vi "test_Outgoing2 Waveforms.vi"(8 "error in (no error)":errorcluster, 11 "DMA Channels Basic Testing in":refnum<class "FPGA Addon DMA Channels Interleaved System Tests.lvclass">) -> (0 "error out":errorcluster, 3 "DMA Channels Basic Testing out":refnum<class "FPGA Addon DMA Channels Interleaved System Tests.lvclass">)   [LabVIEW 2020, in "FPGA Addon DMA Channels Interleaved System Tests.lvclass"]
uses:
  FPGA Addon DMA Channels Interleaved System Tests.lvclass
  FPGA Addon Test Class/FPGA Addon Test Class.lvclass
panel:
  out "Waveform 2":waveform(dbl)(graph)
  out "Waveform 1":waveform(dbl)(graph)
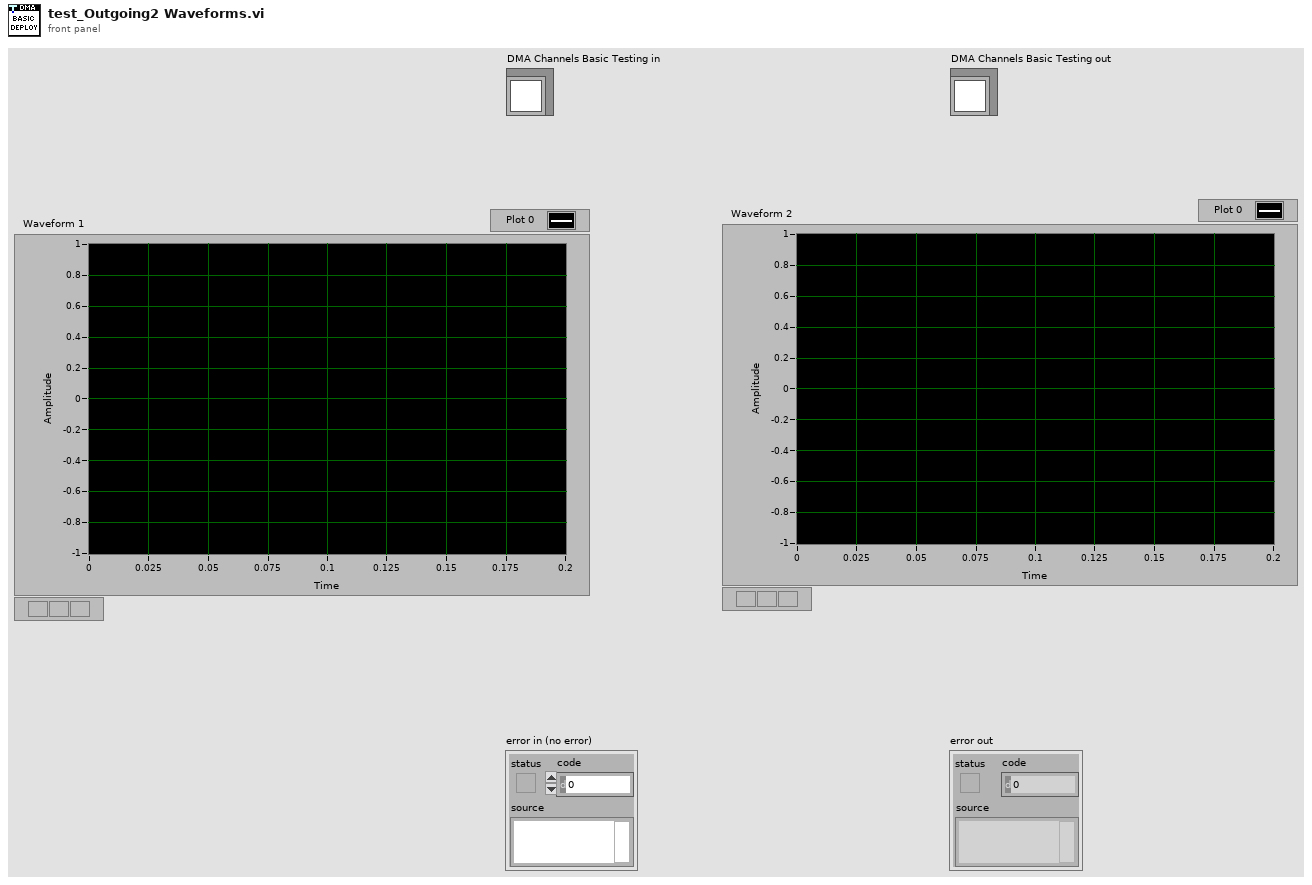
[diagram p1: front panel]
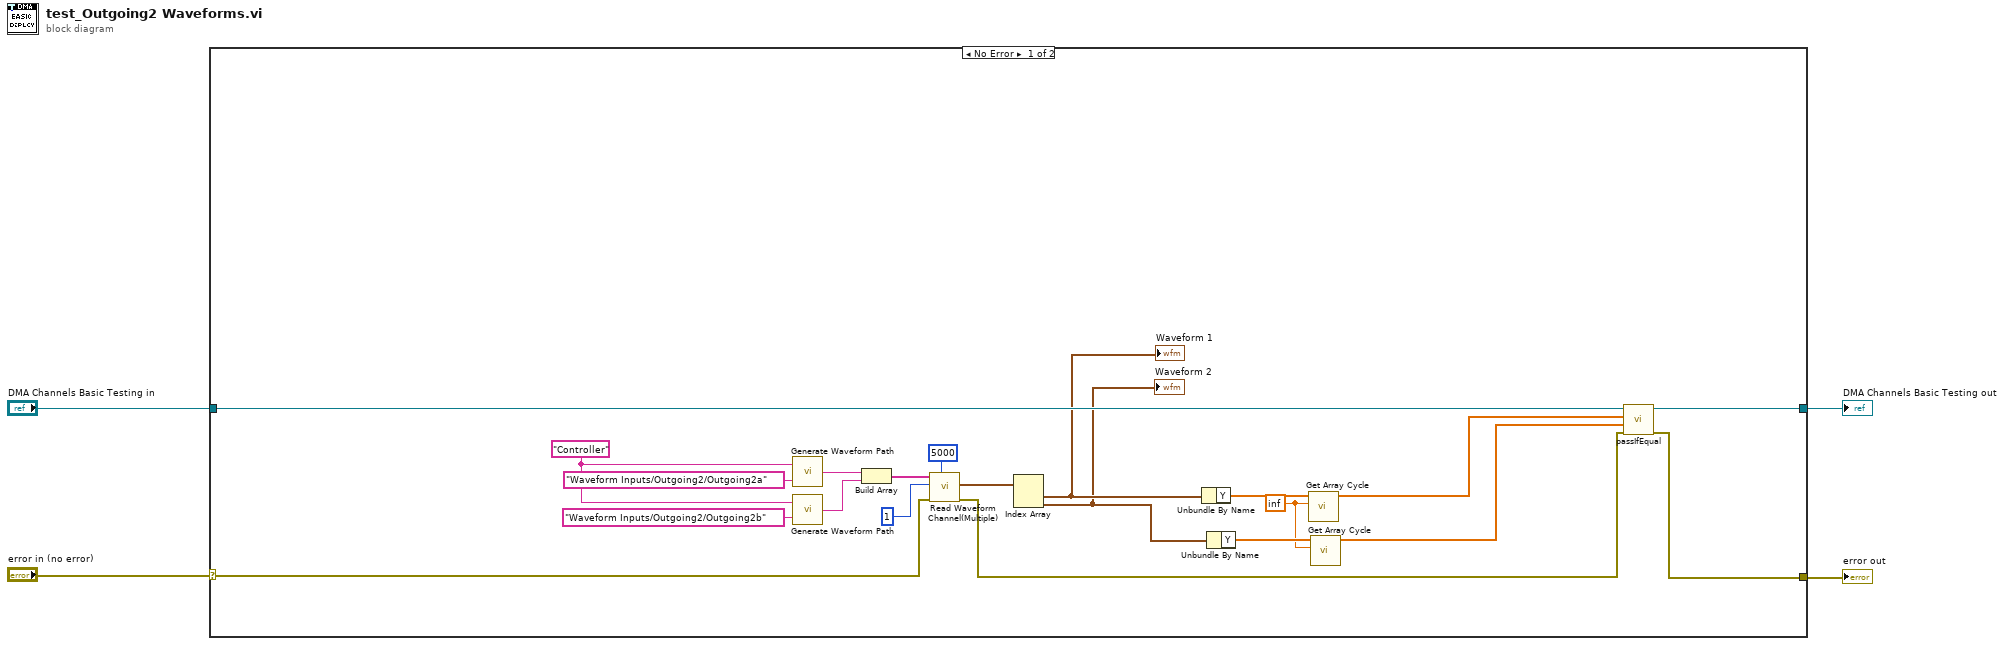
[diagram p0: block diagram]
diagram:
  n1 = case shown="No Error" "error in (no error)" {
    selector: "error in (no error)" -> [w21 w26]
    tunnel: "DMA Channels Basic Testing in" -> [w25 w27]
    tunnel: [w23 w27] -> w1
    tunnel: [w24 w26] -> w3
    frame No Error {
      w8 = "Controller" ("Target Name")
      w15 = inf ("Marker")
      n2 = call "Generate Waveform Path.vi"("Relative Waveform Path"="Waveform Inputs/Outgoing2/Outgoing2a", "Target Name"=w8) -> ("Waveform Path Out"=w7:string)
      n3 = call "Generate Waveform Path.vi"("Relative Waveform Path"="Waveform Inputs/Outgoing2/Outgoing2b", "Target Name"=w8) -> ("Waveform Path Out"=w6:string)
      n4 = Build Array(w7, w6) -> (w5:string[])
      n5 = call "Read Waveform Channel(Multiple).vi"("Timeout"=5000, "error in (no error)"=w21, "Number of Reads"=1, "Waveform Paths in"=w5) -> ("error out"=w19:errorcluster, "Waveform Data"=w22:waveform(dbl)[])  [unwired: 5 in, 1 out]
      n6 = Index Array(array=w22) -> (element #1=w12:waveform(dbl), element #2=w11:waveform(dbl))  [unwired: 2 in]
      "Waveform 1" <- w12
      "Waveform 2" <- w11
      n7 = Unbundle By Name(w12) -> ("Y"=w17:dbl[])
      n8 = Unbundle By Name(w11) -> ("Y"=w16:dbl[])
      n9 = call "Get Array Cycle.vi"("Marker"=w15, "Array Samples"=w17) -> ("Array"=w14:dbl[])  [unwired: 8 in, 1 out]
      n10 = call "Get Array Cycle.vi"("Marker"=w15, "Array Samples"=w16) -> ("Array"=w13:dbl[])  [unwired: 8 in, 1 out]
      n11 = call-dynamic "passIfEqual.vi"("error in (no error)"=w19, "y"=w13, "x"=w14, "TestCase in"=w25) -> ("error out"=w24:errorcluster, "TestCase out"=w23:refnum<class "FPGA Addon DMA Channels Interleaved System Tests.lvclass">)  [unwired: 6 in]
    }
    frame Error {
    }
  }
  "error out" <- w3
  "DMA Channels Basic Testing out" <- w1
